vi "TextBoxLogCtrlMgr.Clear.vi"(10 "error in (no error)":errorcluster, 11 "TextBoxLogCtrlMgr in":refnum<class "TextBoxLogCtrlMgr.lvclass">) -> (2 "error out":errorcluster, 3 "TextBoxLogCtrlMgr out":refnum<class "TextBoxLogCtrlMgr.lvclass">)   [LabVIEW 2024, in "EQMF.lvlib" / "String Utils.lvlib" / "TextBoxLogCtrlMgr.lvclass"]
uses:
  TextBoxLogCtrlMgr.lvclass
  TextBoxLogCtrlMgr.lvclass/TextBoxLogCtrlMgr.ctl
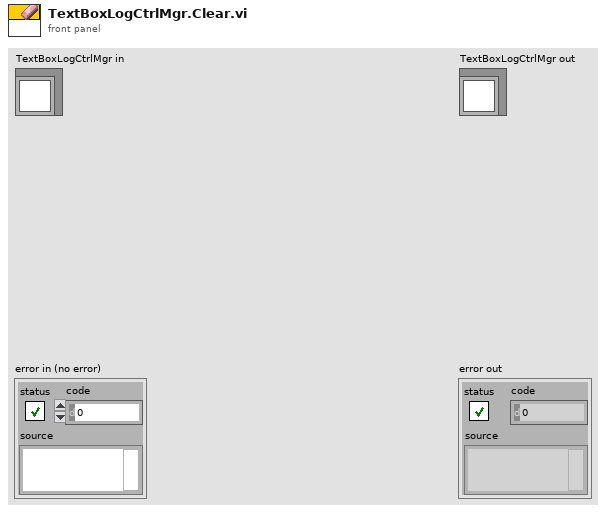
[diagram p1: front panel]
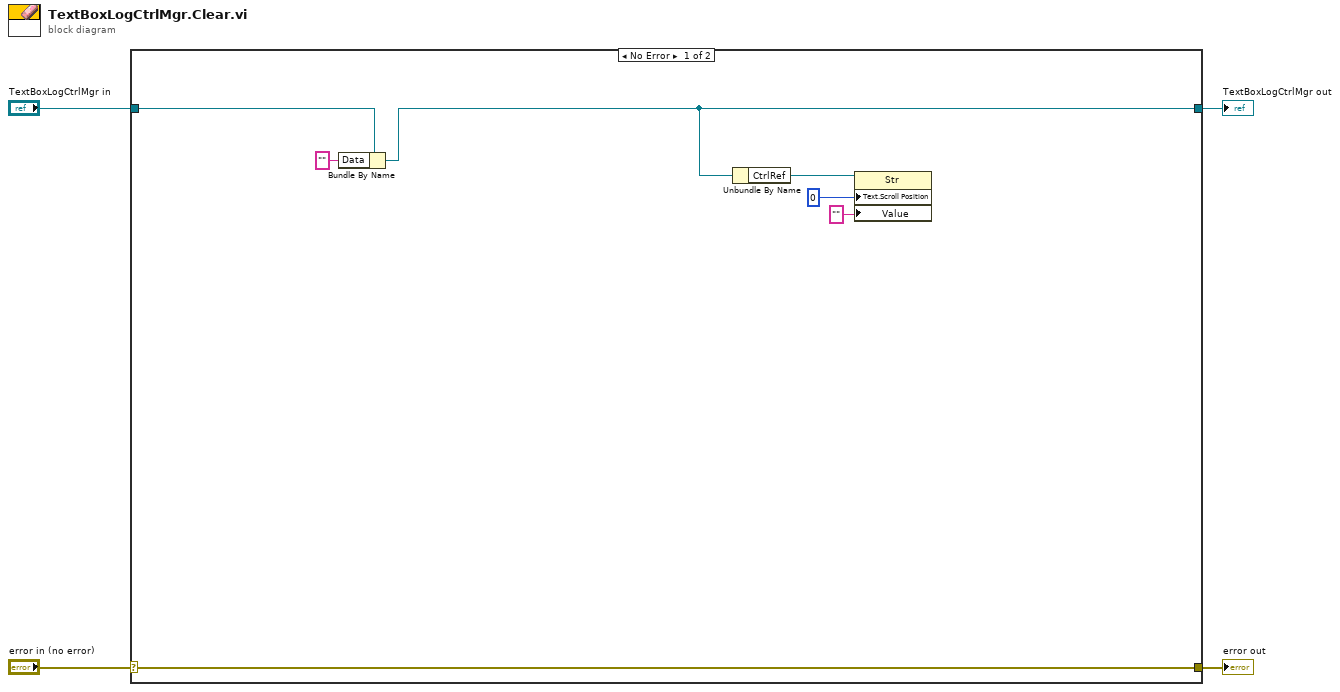
[diagram p0: block diagram]
diagram:
  n1 = case shown="No Error" "error in (no error)" {
    selector: "error in (no error)" -> [w11 w13]
    tunnel: [w11 w13] -> w3
    tunnel: [w8 w12] -> w1
    tunnel: "TextBoxLogCtrlMgr in" -> [w9 w12]
    frame No Error {
      n2 = Bundle By Name(cluster=w9, "Data"="") -> (w8:refnum<class "TextBoxLogCtrlMgr.lvclass">)
      n3 = Unbundle By Name(w8) -> ("CtrlRef"=w10:refnum<vi>)
      n4 = property class="Str"(reference=w10, "Text.Scroll Position"=u32 0, "Value"="") -> ()  [unwired: 1 in, 2 out]
    }
    frame Error {
    }
  }
  "error out" <- w3
  "TextBoxLogCtrlMgr out" <- w1
